vi "WiringPi_PWMWrite.vi"(7 "Value":u16, 8 "error in (no error)":errorcluster, 11 "WiringPi GPIO":T1=7 items=["SDA(I2C)-3"=8, "SCL(I2C)-5"=9, "MOSI(SPI)-19"=12, "MISO(SPI)-21"=13, "SCLK(SPI)-23"=14, "GPIO2-13"=2, "GPIO3-15"=3, "GPIO4-16"=4, "GPIO5-18"=5, "GPIO6-22"=6, "GPIO7-7"=7, "GPIO21-29"=21, "GPIO22-31"=22, "GPIO25-37"=25, "GPIO27-36"=27, "GPIO26(PWM0)-32"=26, "GPIO1(PWM0-12)"=1, "GPIO23(PWM1)-14"=23, "GPIO24(PWM1)-35"=24, "TXD(UART)-8"=15, "RXD(UART)-10"=16, "GPIO10(CE0-SPI)-24"=10, "GPPI11(CE1)-SPI)-26"=11, "GPIO28(PCM_DIN)36"=28, "GPIO29(PCM_DOUT)40"=29]) -> (0 "error out":errorcluster)   [LabVIEW 2014, in "QwaveSys Raspberry Pi Library.lvlib"]
uses:
  QwaveSys Raspberry Pi Library.lvlib
  WiringPi GPIO TypeDef.ctl
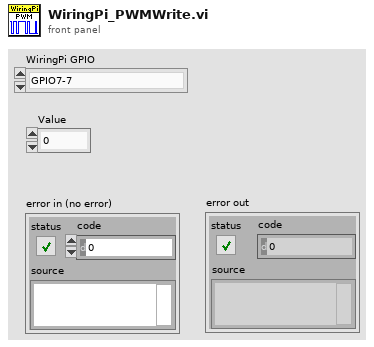
[diagram p1: front panel]
types:
  T1 = typedef "QwaveSys Raspberry Pi Library.lvlib/WiringPi GPIO TypeDef.ctl" = u8
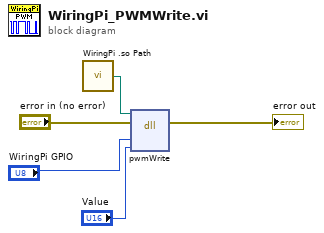
[diagram p0: block diagram]
diagram:
  n1 = call "WiringPi .so Path.vi"() -> ("WiringPi .so Path"=w2:path)  [unwired: 5 in]
  n2 = dll-call lib="libwiringPi.so" fn="pwmWrite"(path in=w2, error in="error in (no error)", "pin"="WiringPi GPIO", "value"="Value") -> (error out=→"error out":errorcluster)  [unwired: 4 in, 1 out]
